vi "Main.vi"() -> ()   [LabVIEW 2018]
panel:
  in  "STOP":bool
  out "Obavestenja":string
  out "SpO2":dbl
  out "Aktivni rezim":bool
  out "Trenutni broj otkucaja u minuti":i32
  in  "Trajanje intervala merenja pulsa (s)":i32
  in  "Start":bool
  in  "Zadatak":enum16{"Sedenje", "Hodanje", "Trcanje"}(ring)
  out "Prikaz PS":dbl(graph)
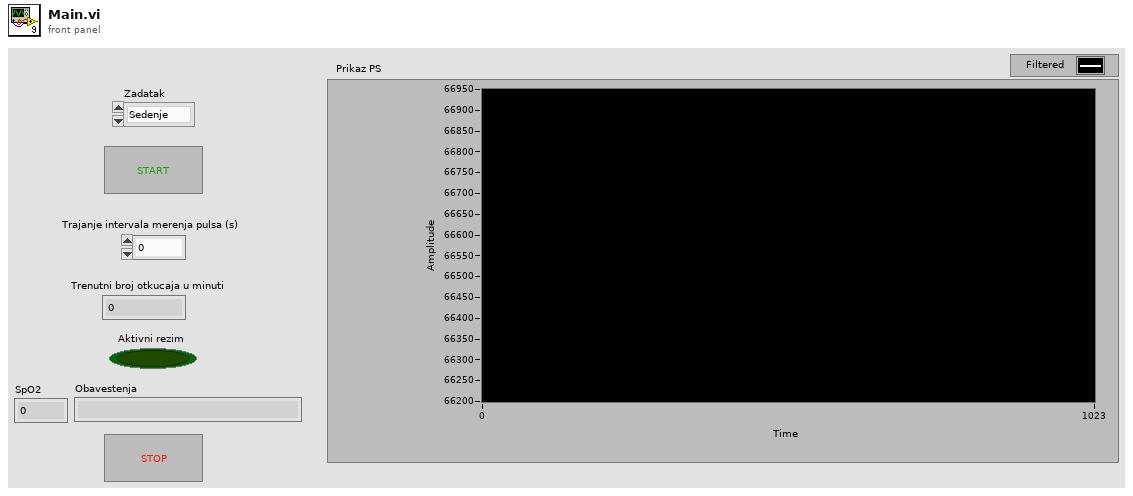
[diagram p1: front panel]
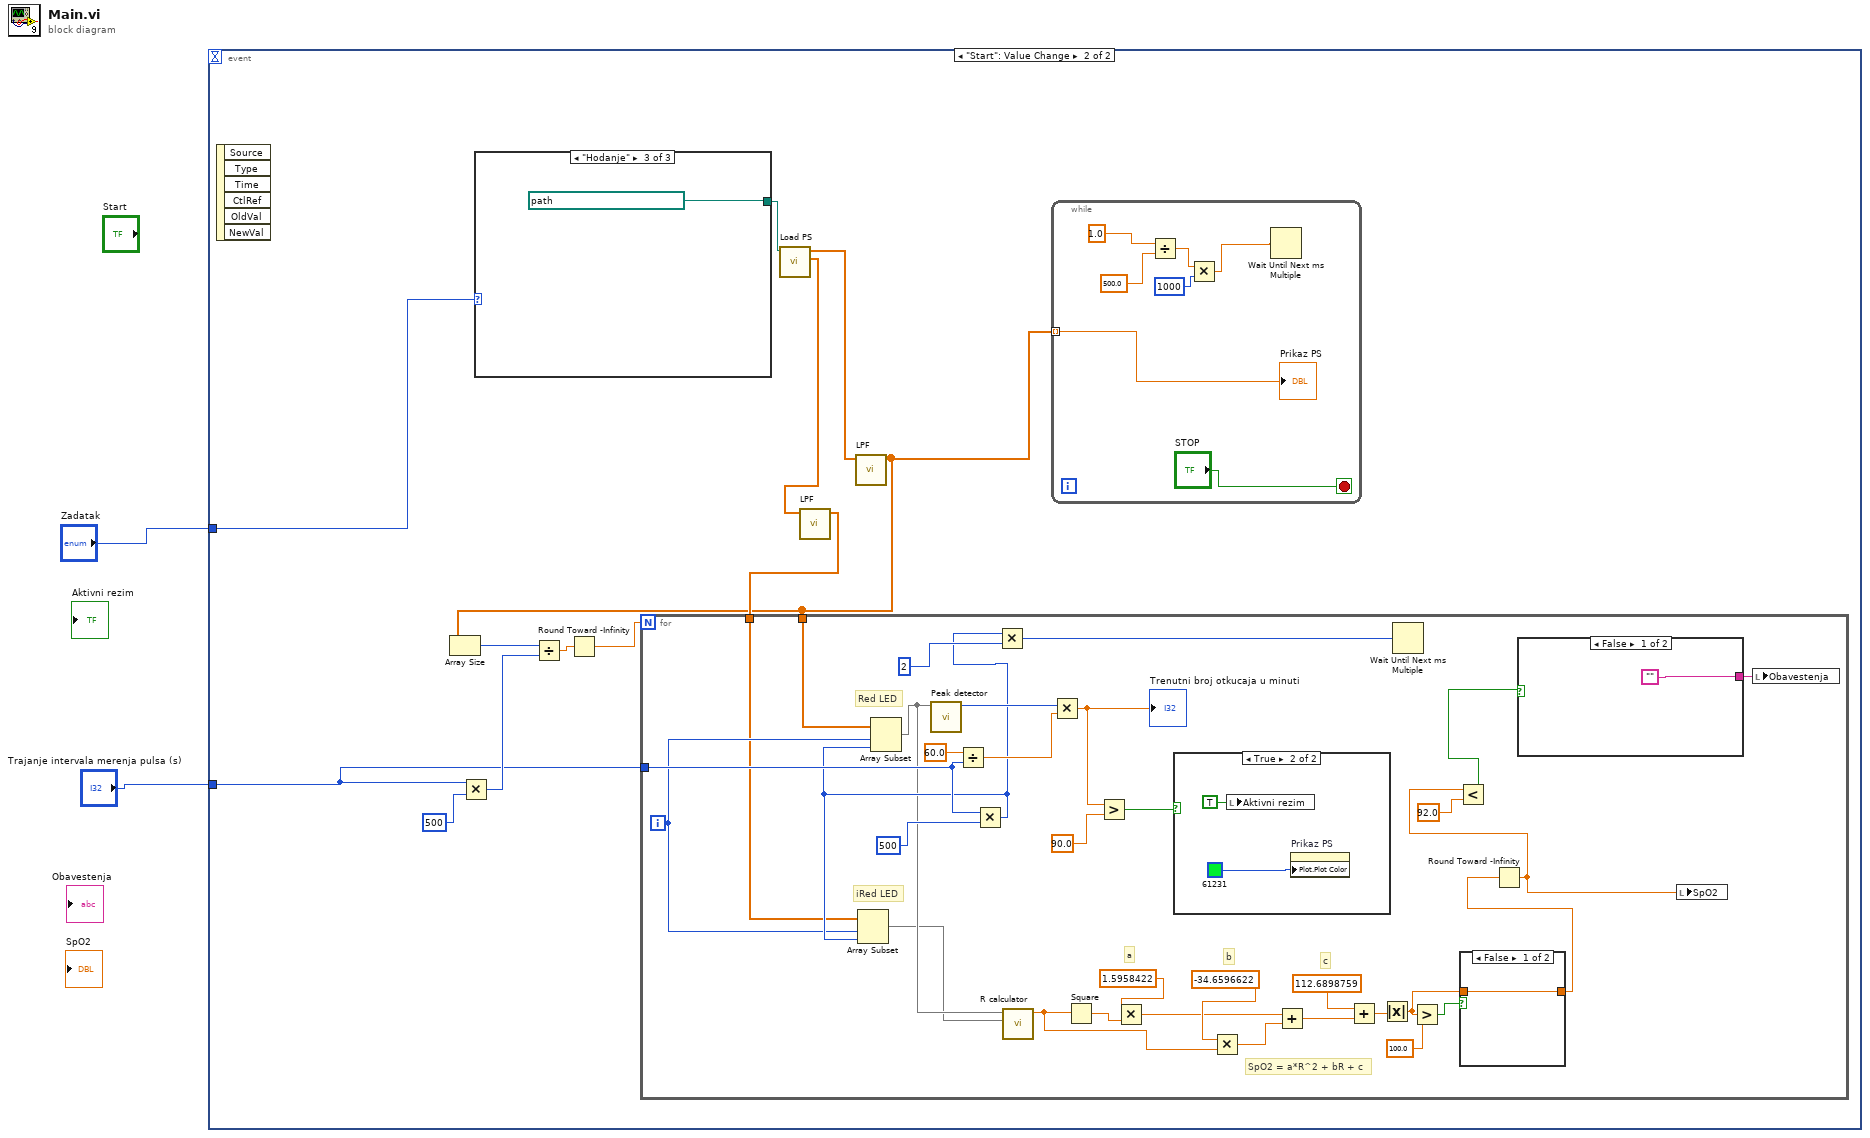
[diagram p0: block diagram]
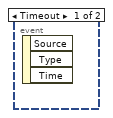
[diagram p2: hidden frame]
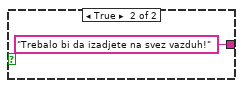
[diagram p3: hidden frame]
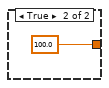
[diagram p4: hidden frame]
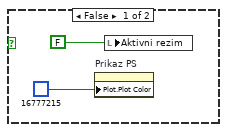
[diagram p5: hidden frame]
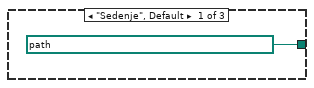
[diagram p6: hidden frame]
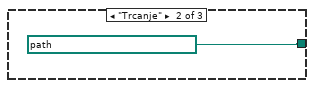
[diagram p7: hidden frame]
diagram:
  n1 = event shown="[1] \"Start\": Value Change" {
    selector: _ -> [_ _]
    dyn-events: _ -> [_ _]
    timeout: _ -> [_ _]
    tunnel: "Zadatak" -> [_ w12]
    tunnel: "Trajanje intervala merenja pulsa (s)" -> [_ w6]
    event Timeout {
      n2 = event-data() -> ()  [unwired: 1 in, 3 out]
    }
    event "Start": Value Change {
      n3 = event-data() -> ()  [unwired: 1 in, 6 out]
      n4 = Multiply(x=w6, y=500) -> (x*y=w11:i32)
      n5 = case shown="\"Hodanje\"" w12 {
        tunnel: [path "C:/Users/djoco/OneDrive/Desktop/Fakultet/4. Godina/8. Semestar/Biomedicinsko inženjerstvo u kognitivnim neuronaukama/Projekat/Data/s10_sit.csv" path "C:/Users/djoco/OneDrive/Desktop/Fakultet/4. Godina/8. Semestar/Biomedicinsko inženjerstvo u kognitivnim neuronaukama/Projekat/Data/s10_run.csv" path "C:/Users/djoco/OneDrive/Desktop/Fakultet/4. Godina/8. Semestar/Biomedicinsko inženjerstvo u kognitivnim neuronaukama/Projekat/Data/s10_sit.csv"] -> w13
        frame "Sedenje", Default {
        }
        frame "Trcanje" {
        }
        frame "Hodanje" {
        }
      }
      n6 = call "Load PS.vi"("Path"=w13) -> ("Array"=w5:dbl[], "Array 2"=w14:dbl[])  [unwired: 9 in]
      n7 = call "LPF.vi"("Subset 3"=w5) -> ("Filtered X"=w4:dbl[])  [unwired: 10 in]
      n8 = call "LPF.vi"("Subset 3"=w14) -> ("Filtered X"=w3:dbl[])  [unwired: 10 in]
      n9 = Array Size(array=w3) -> (size(s)=w7:i32)
      n10 = Divide(x=w7, y=w11) -> (x/y=w8:dbl)
      n11 = Round Toward -Infinity(1:w8) -> (0:w9:dbl)
      n12 = for {
        N: w9 -> [_]
        tunnel: w6 -> [w48]
        tunnel: w3 -> [w47]
        tunnel: w4 -> [w41]
        i -> [w42]
        # "c"
        # "b"
        # "a"
        # "SpO2 = a*R^2 + bR + c"
        # "iRed LED"
        # "Red LED"
        n13 = Divide(x=60.0, y=w48) -> (x/y=w49:dbl)
        n14 = Multiply(x=w48, y=500) -> (x*y=w43:i32)
        n15 = Array Subset(array=w41, index=w42, length=w43) -> (w39:dbl[])
        n16 = Array Subset(array=w47, index=w42, length=w43) -> (w40:dbl[])
        n17 = call "Peak detector.vi"("Filtered X"=w40) -> ("Numeric"=w54:i32)  [unwired: 10 in]
        n18 = Multiply(x=w43, y=2) -> (x*y=w51:i32)
        n19 = call "R calculator.vi"("Filtered X"=w39, "Filtered X 2"=w40) -> ("Numeric"=w35:dbl)  [unwired: 9 in]
        n20 = Multiply(x=w54, y=w49) -> (x*y=w46:dbl)
        "Trenutni broj otkucaja u minuti" <- w46
        n21 = Square(x=w35) -> (x^2=w37:dbl)
        n22 = Greater?(x=w46, y=90.0) -> (0:w44:bool)
        n23 = Multiply(x=1.5958422, y=w37) -> (x*y=w34:dbl)
        n24 = case shown="True" w44 {
          frame False {
            n25 = property on="Prikaz PS" class="WFChart (strict)"("Plot.Plot Color"=u32 16777215) -> ()  [unwired: 2 in, 2 out]
            n26 = local write "Aktivni rezim"(FALSE) -> ()
          }
          frame True {
            n27 = local write "Aktivni rezim"(TRUE ("Aktivni rezim")) -> ()
            n28 = property on="Prikaz PS" class="WFChart (strict)"("Plot.Plot Color"=u32 61231) -> ()  [unwired: 2 in, 2 out]
          }
        }
        n29 = Multiply(x=-34.6596622, y=w35) -> (x*y=w33:dbl)
        n30 = Add(x=w34, y=w33) -> (x+y=w31:dbl)
        n31 = Add(x=112.6898759, y=w31) -> (x+y=w30:dbl)
        n32 = Absolute Value(x=w30) -> (abs(x)=w23:dbl)
        n33 = Wait Until Next ms Multiple(millisecond multiple=w51) -> ()  [unwired: 1 out]
        n34 = Greater?(x=w23, y=100.0) -> (0:w28:bool)
        n35 = case shown="False" w28 {
          tunnel: [w57 100.0 ("y")] -> w22
          tunnel: w23 -> [w57 _]
          frame False {
          }
          frame True {
          }
        }
        n36 = Round Toward -Infinity(1:w22) -> (0:w24:dbl)
        n37 = Less?(x=w24, y=92.0) -> (x < y?=w26:bool)
        n38 = case shown="False" w26 {
          tunnel: ["" "Trebalo bi da izadjete na svez vazduh!"] -> w25
          frame False {
          }
          frame True {
          }
        }
        n39 = local write "SpO2"(w24) -> ()
        n40 = local write "Obavestenja"(w25) -> ()
      }
      n41 = while {
        tunnel: w3 -> [w21] mode=indexing
        stop <- "STOP" stop-if-true
        n42 = Divide(x=1.0, y=500.0) -> (x/y=w18:dbl)
        n43 = Multiply(x=w18, y=1000) -> (x*y=w16:dbl)
        n44 = Wait Until Next ms Multiple(millisecond multiple=w16) -> ()  [unwired: 1 out]
        "Prikaz PS" <- w21
      }
    }
  }
